vi "IRISS V2 Get XYZ Out.vi"(5 "Left or Right Arm":i32(ring)=1 items=["Left Arm", "Right Arm"]) -> (0 "grasp":dbl, 1 "XYZ Out Posit":dbl[](array[numeric]))   [LabVIEW 2016]
uses:
  EyeRobotDLL.dll
panel:
  out "roll":dbl
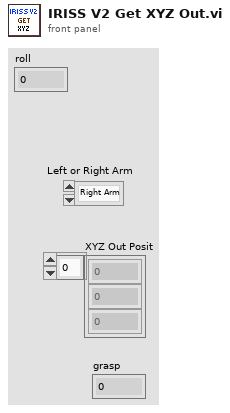
[diagram p1: front panel]
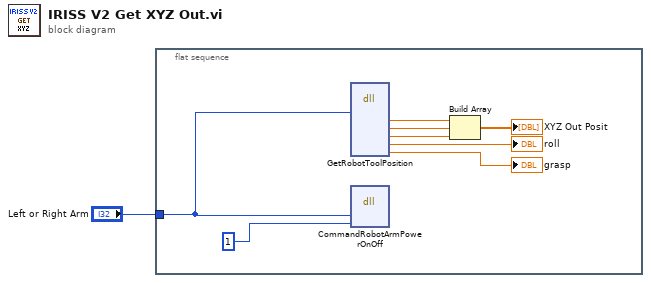
[diagram p0: block diagram]
diagram:
  n1 = flat-sequence {
    tunnel: "Left or Right Arm" -> [w3]
    frame #0 {
      n2 = dll-call lib="D:/Kevin/IRISS V2 dev/Host Demo/Functions/EyeRobotDLL.dll" fn="GetRobotToolPosition"("id"=w3) -> ("x"=w8:dbl, "y"=w6:dbl, "z"=w7:dbl, "roll"=→"roll":dbl, "grasp"=→"grasp":dbl)  [unwired: 10 in, 2 out]
      n3 = dll-call lib="D:/Kevin/IRISS V2 dev/Host Demo/Functions/EyeRobotDLL.dll" fn="CommandRobotArmPowerOnOff"("id"=w3, "OnOff"=1) -> ()  [unwired: 6 in, 2 out]
      n4 = Build Array(w8, w6, w7) -> (→"XYZ Out Posit":dbl[])
    }
  }
